vi "File_Facade.vi"(0 "Data In":T4, 2 "Display State In":T2, 3 "Container State":T3) -> (6 "Data Out":T4, 7 "Display State Out":T2, 8 "Action":T1)   [LabVIEW 2022 SP3, in "File Tree.xctl"]
uses:
  File Tree.xctl
  File_Data.ctl
  <vilib>/_xctls/Container State.ctl
  File_State.ctl
  <vilib>/_xctls/Action.ctl
  <vilib>/_xctls/XControlSupport.lvlib
  <vilib>/Platform/browser.llb/Open URL in Default Browser (string).vi
panel:
  in  "Tree":string(tree)
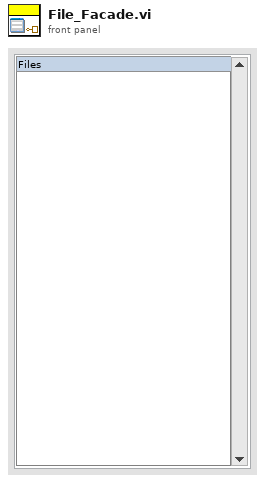
[diagram p1: front panel]
types:
  T1 = typedef "XControlSupport.lvlib/Action.ctl" = cluster{"Data Changed?":bool, "State Changed?":bool, "Action Name":string}
  T2 = typedef "File Tree.xctl/File_State.ctl" = cluster{"Numeric":dbl}
  T3 = typedef "XControlSupport.lvlib/Container State.ctl" = cluster{"Indicator?":bool, "Run Mode?":bool, " Refnum":refnum<vi>}
  T4 = typedef "File Tree.xctl/File_Data.ctl" = path
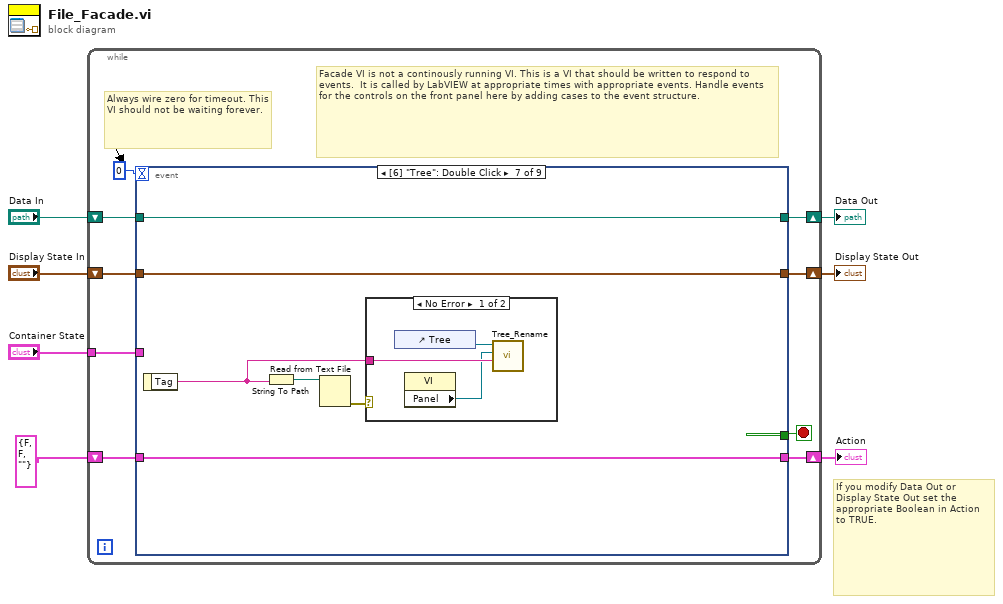
[diagram p0: block diagram]
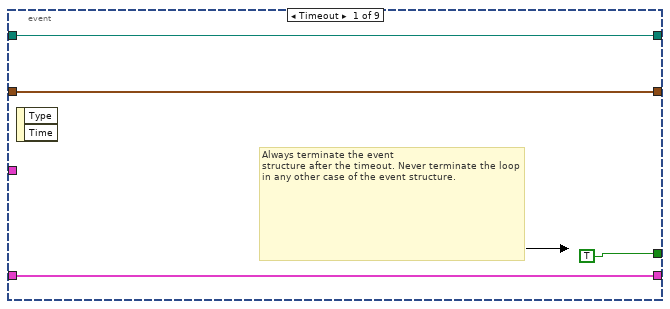
[diagram p2: hidden frame]
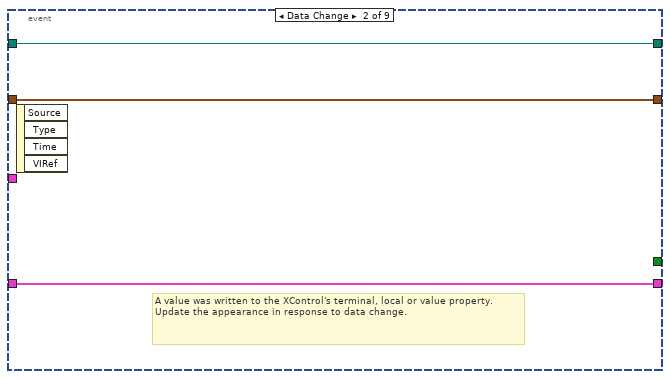
[diagram p3: hidden frame]
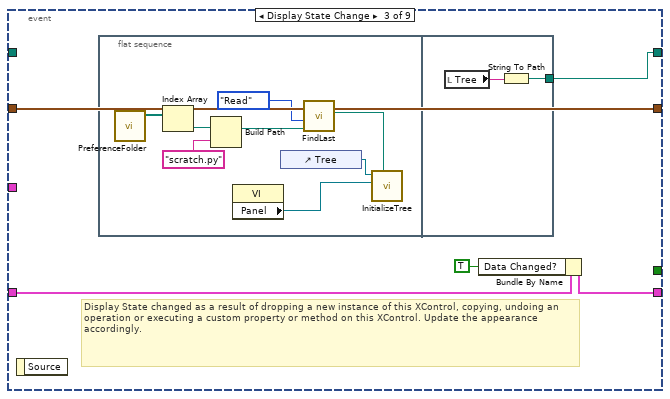
[diagram p4: hidden frame]
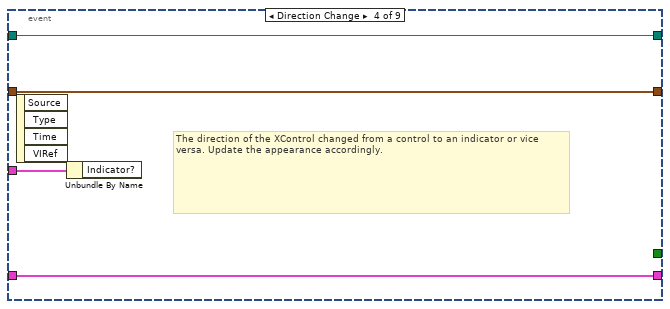
[diagram p5: hidden frame]
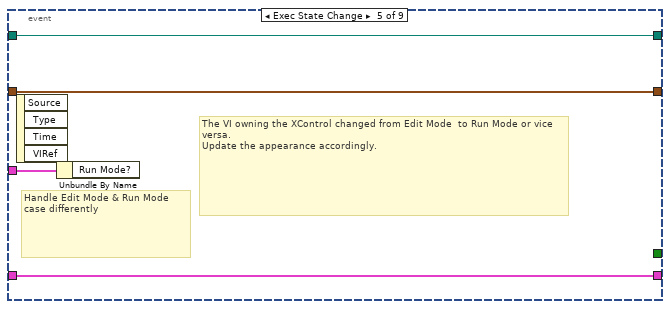
[diagram p6: hidden frame]
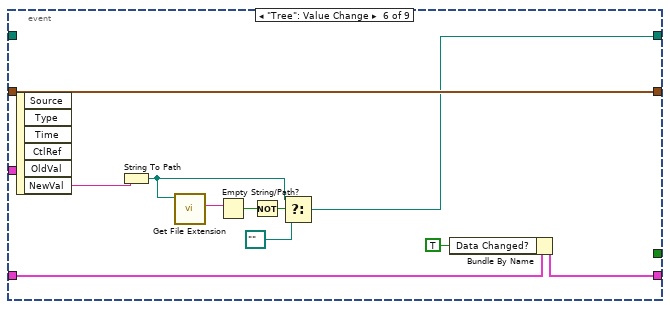
[diagram p7: hidden frame]
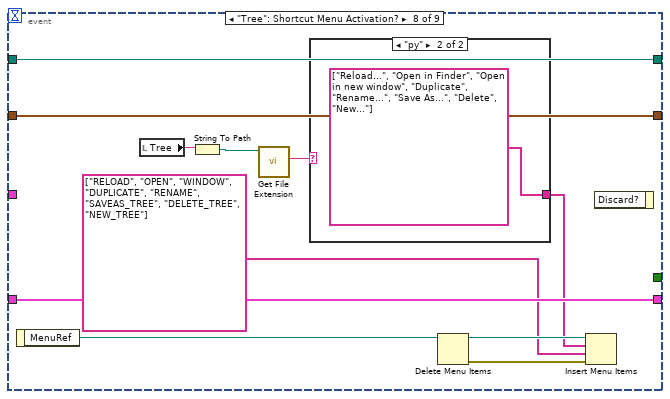
[diagram p9: hidden frame]
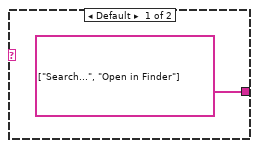
[diagram p10: hidden frame]
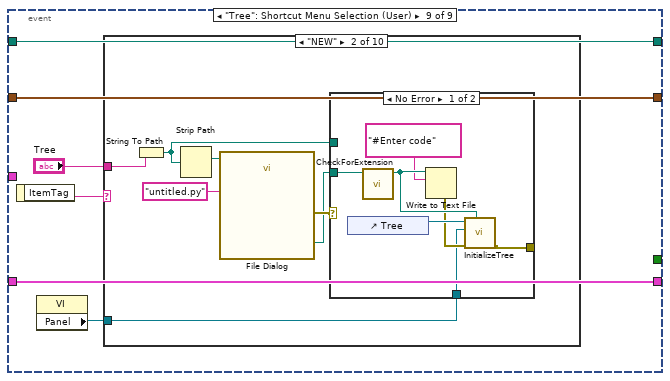
[diagram p11: hidden frame]
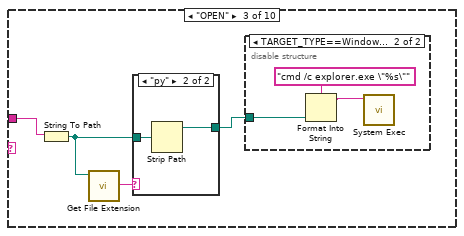
[diagram p14: hidden frame]
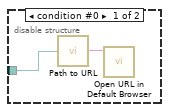
[diagram p15: hidden frame]
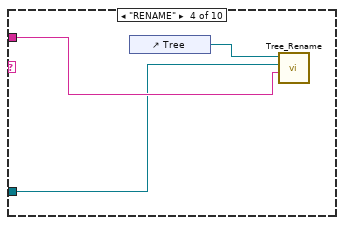
[diagram p17: hidden frame]
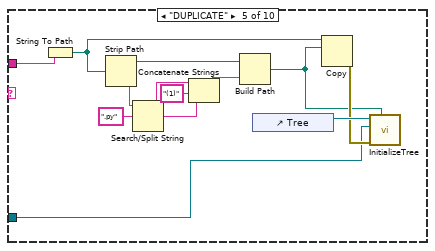
[diagram p18: hidden frame]
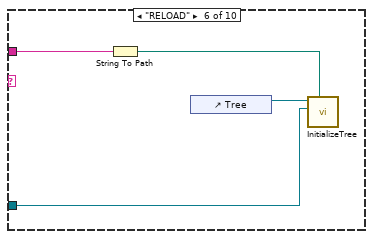
[diagram p19: hidden frame]
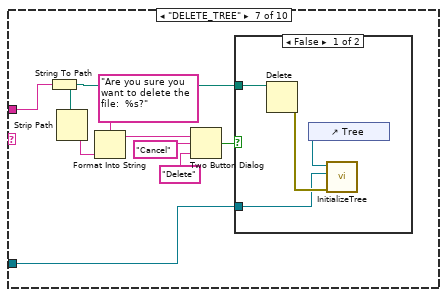
[diagram p20: hidden frame]
diagram:
  # "If you modify Data Out or\nDisplay State Out set the\nappropriate Boolean in Action\nto TRUE."
  n1 = while {
    shift-right: [w15] -> w4
    shift-left: "Display State In" -> [w16]
    tunnel: "Container State" -> [w12]
    shift-right: [w10] -> w7
    shift-left: "Data In" -> [w11]
    shift-right: [w8] -> w2
    shift-left: T1 {"Data Changed?"=FALSE, "State Changed?"=FALSE, "Action Name"=""} ("Action") -> [w9]
    stop <- w14 stop-if-true
    # "Facade VI is not a continously running VI. This is a VI that should be written to respond to events.  It is called by LabVIEW at appropriate times with appropriate events. Handle events for the controls on the front panel here by adding cases to the event structure."
    # "Always wire zero for timeout. This\nVI should not be waiting forever."
    n2 = event shown="[6] \"Tree\": Double Click" {
      selector: _ -> [_ _ _ _ _ _ _ _ _]
      dyn-events: _ -> [_ _ _ _ _ _ _ _ _]
      timeout: 0 -> [_ _ _ _ _ _ _ _ _]
      tunnel: w16 -> [w18 w22 w28 w41 w45 w57 w63 w77 w85]
      tunnel: [w18 w22 w28 w41 w45 w57 w63 w77 w85] -> w15
      tunnel: [TRUE _ _ _ _ _ _ _ _] -> w14
      tunnel: w12 -> [_ _ _ w42 w46 _ _ _ _]
      tunnel: w11 -> [w17 w23 _ w40 w44 _ w62 w76 w84]
      tunnel: [w17 w23 w24 w40 w44 w47 w62 w76 w84] -> w10
      tunnel: [w19 w21 w27 w39 w43 w55 w61 w75 w83] -> w8
      tunnel: w9 -> [w19 w21 w26 w39 w43 w54 w61 w75 w83]
      event Timeout {
        # "Always terminate the event\nstructure after the timeout. Never terminate the loop in any other case of the event structure."
        n3 = event-data() -> ()  [unwired: 1 in, 2 out]
      }
      event Data Change {
        # "A value was written to the XControl's terminal, local or value property.\nUpdate the appearance in response to data change."
        n4 = event-data() -> ()  [unwired: 1 in, 4 out]
      }
      event Display State Change {
        # "Display State changed as a result of dropping a new instance of this XControl, copying, undoing an operation or executing a custom property or method on this XControl. Update the appearance accordingly."
        n5 = event-data() -> ()  [unwired: 1 in, 1 out]
        n6 = flat-sequence {
          tunnel: [w37] -> w24
          frame #0 {
            n7 = call "PreferenceFolder.vi"() -> ("pythonCodes"=w33:path[])  [unwired: 4 in, 7 out]
            n8 = Index Array(array=w33) -> (element=w34:path)  [unwired: 1 in]
            n9 = Build Path(base path=w34, name or relative path="scratch.py" ("Python Code")) -> (appended path=w35:path)
            n10 = property class="VI"() -> ("Panel"=w29:refnum<vi>)  [unwired: 2 in, 2 out]
            n11 = control-ref of="Tree"() -> (w32:refnum<vi>)
            n12 = call "FindLast.vi"("default"=w35, "Task"=enum16{"Save", "Read"}."Read") -> ("path"=w36:path)  [unwired: 9 in]
            n13 = call "InitializeTree.vi"("Selected File"=w36, "Panel"=w29, "TreeControl in"=w32) -> ()  [unwired: 7 in, 2 out]
          }
          frame #1 {
            n14 = local read "Tree"() -> (w38:string)
            n15 = String To Path(string=w38) -> (path=w37:path)
          }
        }
        n16 = Bundle By Name(cluster=w26, "Data Changed?"=TRUE) -> (w27:T1)
      }
      event Direction Change {
        # "The direction of the XControl changed from a control to an indicator or vice versa. Update the appearance accordingly."
        n17 = event-data() -> ()  [unwired: 1 in, 4 out]
        n18 = Unbundle By Name(w42) -> ()  [unwired: 1 out]
      }
      event Exec State Change {
        # "The VI owning the XControl changed from Edit Mode  to Run Mode or vice versa.\nUpdate the appearance accordingly."
        # "Handle Edit Mode & Run Mode\ncase differently"
        n19 = event-data() -> ()  [unwired: 1 in, 4 out]
        n20 = Unbundle By Name(w46) -> ()  [unwired: 1 out]
      }
      event "Tree": Value Change {
        n21 = event-data() -> ("NewVal"=w56:string)  [unwired: 1 in, 5 out]
        n22 = String To Path(string=w56) -> (path=w49:path)
        n23 = call <vilib>:"Get File Extension.vi"("file"=w49) -> ("lowercase file extension"=w52:string)  [unwired: 6 in, 4 out]
        n24 = Empty String/Path?(string/path=w52) -> (empty?=w51:bool)
        n25 = Not(x=w51) -> (.not. x?=w50:bool)
        n26 = Select(t=w49, s=w50, f=path "") -> (s? t:f=w47:path)
        n27 = Bundle By Name(cluster=w54, "Data Changed?"=TRUE) -> (w55:T1)
      }
      event "Tree": Double Click {
        n28 = event-data() -> ("Tag"=w59:string)  [unwired: 1 in]
        n29 = String To Path(string=w59) -> (path=w60:path)
        n30 = Read from Text File(file (use dialog)=w60) -> (error out=w58:errorcluster)  [unwired: 3 in, 3 out]
        n31 = case shown="No Error" w58 {
          tunnel: w59 -> [w65 _]
          frame No Error {
            n32 = control-ref of="Tree"() -> (w66:refnum<vi>)
            n33 = property class="VI"() -> ("Panel"=w64:refnum<vi>)  [unwired: 2 in, 2 out]
            n34 = call "Tree_Rename.vi"("Tree in"=w65, "Panel"=w64, "TreeControl in"=w66) -> ()  [unwired: 9 in]
          }
          frame Error {
          }
        }
      }
      event "Tree": Shortcut Menu Activation? {
        n35 = event-data() -> ("MenuRef"=w67:refnum<k9>)  [unwired: 1 in]
        n36 = local read "Tree"() -> (w70:string)
        n37 = String To Path(string=w70) -> (path=w69:path)
        n38 = call <vilib>:"Get File Extension.vi"("file"=w69) -> ("lowercase file extension"=w68:string)  [unwired: 6 in, 4 out]
        n39 = case shown="\"py\"" w68 {
          tunnel: [string[] ["Search...", "Open in Finder"] ("L10n_Parent Menus") string[] ["Reload...", "Open in Finder", "Open in new window", "Duplicate", "Rename...", "Save As...", "Delete", "New..."] ("L10n_Parent Menus")] -> w71
          frame Default {
          }
          frame "py" {
          }
        }
        n40 = Delete Menu Items(9:w67) -> (0:w74:errorcluster, 3:w73:refnum<k9>)  [unwired: 3 in]
        n41 = Insert Menu Items(6:w74, 7:string[] ["RELOAD", "OPEN", "WINDOW", "DUPLICATE", "RENAME", "SAVEAS_TREE", "DELETE_TREE", "NEW_TREE"], 8:w71, 9:w73) -> ()  [unwired: 2 in, 3 out]
        n42 = event-data() -> ()  [unwired: 2 in, 1 out]
      }
      event "Tree": Shortcut Menu Selection (User) {
        n43 = event-data() -> ("ItemTag"=w82:string)  [unwired: 1 in]
        n44 = property class="VI"() -> ("Panel"=w80:refnum<vi>)  [unwired: 2 in, 2 out]
        n45 = case shown="\"NEW\"" w82 {
          tunnel: "Tree" -> [_ w87 w100 w113 w115 w129 w133 w146 w161 w174]
          tunnel: w80 -> [_ w86 _ w112 w116 w128 w132 w145 w160 _]
          frame Default {
          }
          frame "NEW" {
            n46 = String To Path(string=w87) -> (path=w92:path)
            n47 = Strip Path(path=w92) -> (stripped path=w91:path)  [unwired: 1 out]
            n48 = call "File Dialog"("start path"=w91, "default name"="untitled.py") -> ("selected path"=w89:path, "error out"=w90:errorcluster)  [unwired: 10 in, 2 out]
            n49 = case shown="No Error" w90 {
              tunnel: w92 -> [_ _]
              tunnel: w89 -> [w99 _]
              tunnel: [w94 _] -> _
              tunnel: w86 -> [w93 _]
              frame No Error {
                n50 = control-ref of="Tree"() -> (w98:refnum<vi>)
                n51 = call "CheckForExtension.vi"("selected path"=w99) -> ("dup file"=w97:path)  [unwired: 10 in]
                n52 = Write to Text File(file (use dialog)=w97, text="#Enter code") -> (error out=w96:errorcluster)  [unwired: 2 in, 2 out]
                n53 = call "InitializeTree.vi"("Selected File"=w97, "error in (no error)"=w96, "Panel"=w93, "TreeControl in"=w98) -> ("error out"=w94:errorcluster)  [unwired: 6 in, 1 out]
              }
              frame Error {
              }
            }
          }
          frame "OPEN" {
            n54 = String To Path(string=w100) -> (path=w103:path)
            n55 = call <vilib>:"Get File Extension.vi"("file"=w103) -> ("lowercase file extension"=w102:string)  [unwired: 6 in, 4 out]
            n56 = case shown="\"py\"" w102 {
              tunnel: [w109 w111] -> w101
              tunnel: w103 -> [w109 w110]
              frame Default {
              }
              frame "py" {
                n57 = Strip Path(path=w110) -> (stripped path=w111:path)  [unwired: 1 out]
              }
            }
            n58 = disable-structure shown="TARGET_TYPE==Windows" {
              disable-tunnel: w101 -> [w105 w106]
              frame condition #0 {
                n59 = call <vilib>:"Path to URL.vi"("path"=w105) -> ("url"=w104:string)
                n60 = call-poly <vilib>:"Open URL in Default Browser.vi"("URL"=w104) -> ()  [unwired: 5 in, 2 out]
              }
              frame condition #1 (active) {
                n61 = Format Into String(format string="cmd /c explorer.exe \"%s\"", w106) -> (resulting string=w108:string)  [unwired: 2 in, 1 out]
                n62 = call <vilib>:"System Exec.vi"("command line"=w108) -> ()  [unwired: 7 in, 4 out]
              }
            }
          }
          frame "RENAME" {
            n63 = control-ref of="Tree"() -> (w114:refnum<vi>)
            n64 = call "Tree_Rename.vi"("Tree in"=w113, "Panel"=w112, "TreeControl in"=w114) -> ()  [unwired: 9 in]
          }
          frame "DUPLICATE" {
            n65 = String To Path(string=w115) -> (path=w127:path)
            n66 = Strip Path(path=w127) -> (stripped path=w126:path, name=w122:string)
            n67 = Search/Split String(string=w122, search string/char (-)=".py") -> (substring before match=w120:string, match + rest of string=w119:string)  [unwired: 1 in, 1 out]
            n68 = Concatenate Strings(w120, "(1)" ("search string/char (-)"), w119) -> (w118:string)
            n69 = Build Path(base path=w126, name or relative path=w118) -> (appended path=w123:path)
            n70 = control-ref of="Tree"() -> (w125:refnum<vi>)
            n71 = Copy(10:w123, 11:w127) -> (0:w124:errorcluster)  [unwired: 3 in, 2 out]
            n72 = call "InitializeTree.vi"("Selected File"=w123, "error in (no error)"=w124, "Panel"=w116, "TreeControl in"=w125) -> ()  [unwired: 6 in, 2 out]
          }
          frame "RELOAD" {
            n73 = String To Path(string=w129) -> (path=w130:path)
            n74 = control-ref of="Tree"() -> (w131:refnum<vi>)
            n75 = call "InitializeTree.vi"("Selected File"=w130, "Panel"=w128, "TreeControl in"=w131) -> ()  [unwired: 7 in, 2 out]
          }
          frame "DELETE_TREE" {
            n76 = String To Path(string=w133) -> (path=w139:path)
            n77 = Strip Path(path=w139) -> (name=w138:string)  [unwired: 1 out]
            n78 = Format Into String(format string="Are you sure you want to delete the file:  %s?", w138) -> (resulting string=w137:string)  [unwired: 2 in, 1 out]
            n79 = Two Button Dialog(message=w137, 1:"Delete" ("T button name (\"OK\")"), 2:"Cancel" ("T button name (\"OK\")")) -> (T button?=w140:bool)
            n80 = case shown="False" w140 {
              tunnel: w139 -> [w144 _]
              tunnel: w132 -> [w141 _]
              frame False {
                n81 = Delete(path (use dialog)=w144) -> (error out=w142:errorcluster)  [unwired: 4 in, 2 out]
                n82 = control-ref of="Tree"() -> (w143:refnum<vi>)
                n83 = call "InitializeTree.vi"("error in (no error)"=w142, "Panel"=w141, "TreeControl in"=w143) -> ()  [unwired: 7 in, 2 out]
              }
              frame True {
              }
            }
          }
          frame "NEW_TREE" {
            n84 = String To Path(string=w146) -> (path=w148:path)
            n85 = call "File Dialog2"("start path"=w148) -> ("selected path"=w149:path, "error out"=w147:errorcluster)  [unwired: 11 in, 2 out]
            n86 = case shown="No Error" w147 {
              tunnel: w145 -> [w153 _]
              tunnel: w149 -> [w151 _]
              frame No Error {
                n87 = call "CheckForExtension.vi"("selected path"=w151) -> ("dup file"=w150:path)  [unwired: 10 in]
                n88 = call <vilib>:"Check if File or Folder Exists.vi"("path"=w151) -> ("file or folder exists?"=w152:bool)  [unwired: 8 in, 2 out]
                n89 = case shown="False" w152 {
                  tunnel: w153 -> [w157 _]
                  tunnel: w150 -> [w156 _]
                  frame False {
                    n90 = call <vilib>:"Create File and Containing Folders.vi"("file path"=w156) -> ("refnum out"=w155:refnum<file>)  [unwired: 9 in, 1 out]
                    n91 = Write to Text File(file (use dialog)=w155, text="#Enter code\n\n") -> ()  [unwired: 2 in, 3 out]
                    n92 = control-ref of="Tree"() -> (w158:refnum<vi>)
                    n93 = call "InitializeTree.vi"("Selected File"=w156, "Panel"=w157, "TreeControl in"=w158) -> ()  [unwired: 7 in, 2 out]
                  }
                  frame True {
                    n94 = One Button Dialog(message="File already exists") -> ()  [unwired: 1 in, 1 out]
                  }
                }
              }
              frame Error {
              }
            }
          }
          frame "SAVEAS_TREE" {
            n95 = String To Path(string=w161) -> (path=w165:path)
            n96 = Strip Path(path=w165) -> (stripped path=w164:path, name=w166:string)
            n97 = call "File Dialog3"("start path"=w164, "default name"=w166) -> ("selected path"=w162:path, "error out"=w163:errorcluster)  [unwired: 10 in, 2 out]
            n98 = case shown="No Error" w163 {
              tunnel: w165 -> [w169 _]
              tunnel: w162 -> [w173 _]
              tunnel: w160 -> [w171 _]
              tunnel: [w170 _] -> _
              frame No Error {
                n99 = control-ref of="Tree"() -> (w172:refnum<vi>)
                n100 = call "CheckForExtension.vi"("selected path"=w173) -> ("dup file"=w168:path)  [unwired: 10 in]
                n101 = Copy(10:w168, 11:w169) -> (0:w167:errorcluster)  [unwired: 3 in, 2 out]
                n102 = call "InitializeTree.vi"("Selected File"=w168, "error in (no error)"=w167, "Panel"=w171, "TreeControl in"=w172) -> ("error out"=w170:errorcluster)  [unwired: 6 in, 1 out]
              }
              frame Error {
              }
            }
          }
          frame "WINDOW" {
            w177 = 128  # call and forget
            n103 = String To Path(string=w174) -> (path=w176:path)
            n104 = vi-ref "MainWindow.vi"() -> (w181:refnum<vi>)
            n105 = property class="VI"(reference=w181) -> ("Name"=w180:string)  [unwired: 1 in, 2 out]
            n106 = Open VI Reference(type specifier VI Refnum (for type only)=refnum<vi> refnum, vi path=w180, options=w177) -> (vi reference=w179:refnum<vi>, error out=w184:errorcluster)  [unwired: 3 in]
            n107 = call-by-ref "Start Asynchronous Call"(reference=w179, error in=w184, "Path"=w176) -> (reference out=w183:refnum<vi>, error out=w182:errorcluster)  [unwired: 11 in]
            n108 = property on="Tree" class="Tree (strict)"("Val(Sgnl)"="" ("Value (Signaling)")) -> ()  [unwired: 2 in, 2 out]
            n109 = Close Reference(reference=w183, error in (no error)=w182) -> ()  [unwired: 1 out]
          }
        }
      }
    }
  }
  "Display State Out" <- w4
  "Data Out" <- w7
  "Action" <- w2
